vi "Configure.vi"(8 "error in (no error)":errorcluster, 11 "Autofocus in":refnum<class "Autofocus.lvclass">) -> (0 "error out":errorcluster, 2 "cancelled?":bool, 3 "Autofocus out":refnum<class "Autofocus.lvclass">)   [LabVIEW 2012, in "Autofocus.lvclass"]
doc: "The configure method configures the details for the RabbitMQ connection, the observers and the mapping script.\n\nIn the derived class, make a call to the parent for setting these parameters."
uses:
  Autofocus.lvclass
  number of subregions.ctl
  <vilib>/Utility/miscctls.llb/LVPointTypeDef.ctl
  Autofocus.lvclass/Autofocus.ctl
  <vilib>/Distrio/Murmex/Murmex/Murmex.lvclass
panel:
  in  "button::ok":bool
  in  "button::configure murmex":bool
  in  "button::cancel":bool
  in  "Tab Control":T1(tab)
  in  "Sample stage component name":string
  in  "Tomo component name":string
  in  "Camera component name":string
  in  "Focus stage component name":string
  in  "Epsilon (HC)":dbl
  in  "Epsilon (GS)":dbl
  in  "Image File Path":path
  in  "Number of subregions":T2 items=["4"=4, "5"=5]
  # "RabbitMQ parameters"
  # "Window position"
  # "Stopping parameters"
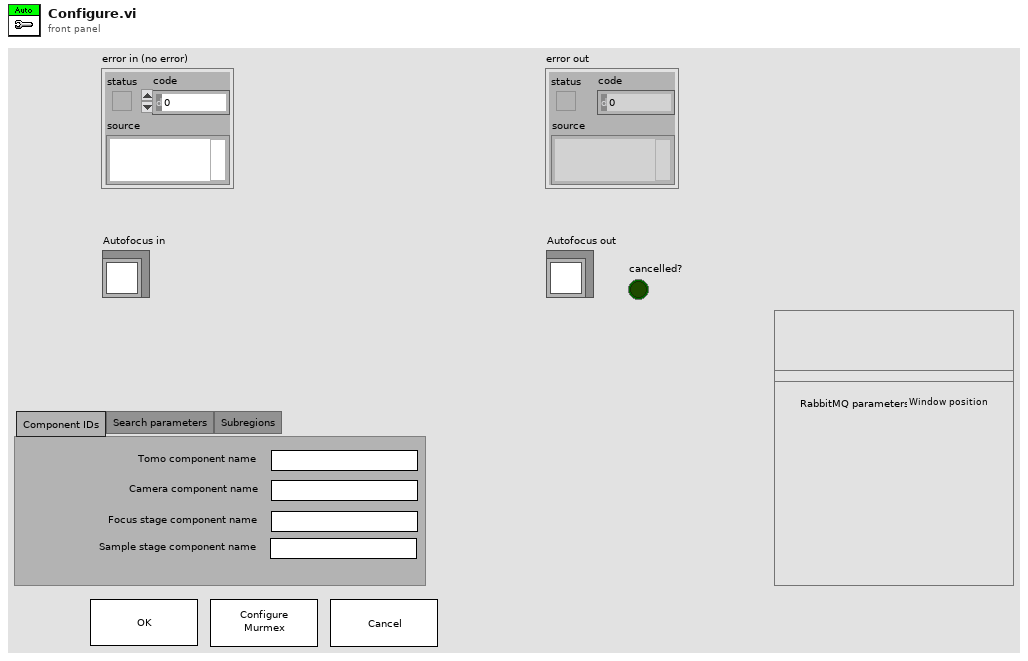
[diagram p1: front panel]
types:
  T1 = enum32{"Component IDs", "Search parameters", "Subregions"}
  T2 = typedef "Autofocus.lvclass/number of subregions.ctl" = i32
  T3 = typedef "LVPointTypeDef.ctl" = cluster{"Horizontal":i16, "Vertical":i16}
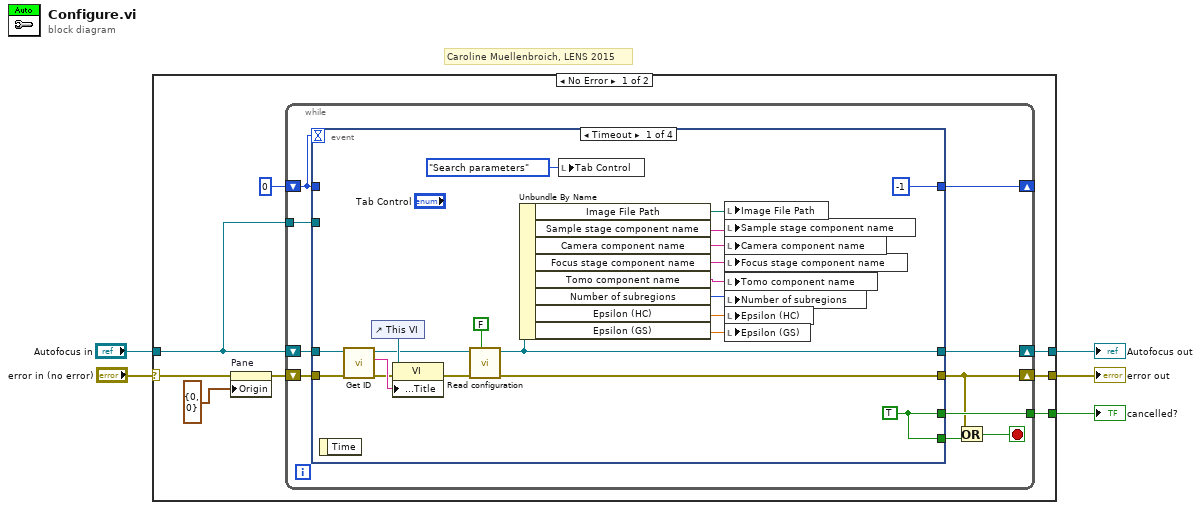
[diagram p0: block diagram]
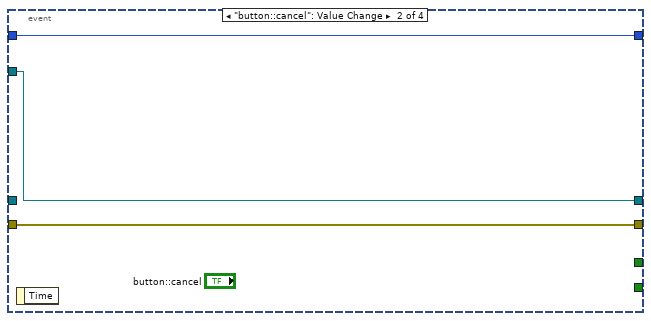
[diagram p2: hidden frame]
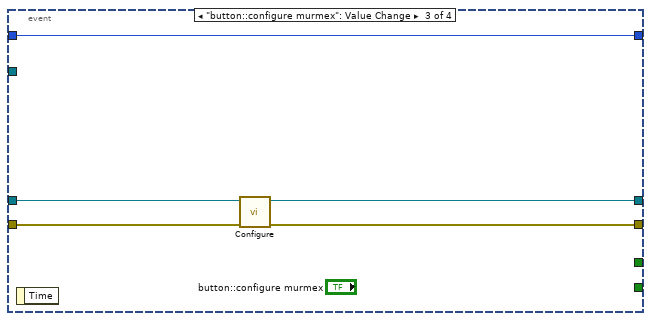
[diagram p3: hidden frame]
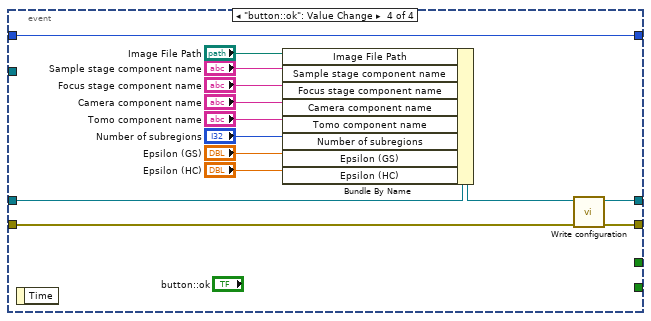
[diagram p4: hidden frame]
diagram:
  # "Caroline Muellenbroich, LENS 2015"
  n1 = case shown="No Error" "error in (no error)" {
    selector: "error in (no error)" -> [w12 w68]
    tunnel: "Autofocus in" -> [w10 w67]
    tunnel: [w8 w68] -> w3
    tunnel: [w7 w67] -> w2
    tunnel: [w6 _] -> w1
    frame No Error {
      n2 = property on="Pane" class="Pane"(error in=w12, "Origin"=T3 {"Horizontal"=0, "Vertical"=0}) -> (error out=w11:errorcluster)  [unwired: 1 in, 1 out]
      n3 = while {
        shift-right: [w18] -> w7
        shift-left: w10 -> [w20]
        shift-right: [w15] -> w8
        shift-left: w11 -> [w21]
        tunnel: w10 -> [w23]
        shift-right: [w19] -> _
        shift-left: 0 -> [w22]
        tunnel: [w17] -> w6
        stop <- w16 stop-if-true
        n4 = event shown="[0] Timeout" {
          selector: _ -> [_ _ _ _]
          dyn-events: _ -> [_ _ _ _]
          timeout: w22 -> [_ _ _ _]
          tunnel: w23 -> [_ w45 _ _]
          tunnel: w22 -> [_ w46 w48 w61]
          tunnel: w21 -> [w42 w47 w52 w64]
          tunnel: w20 -> [w41 _ w50 w63]
          tunnel: [-1 w46 w48 w61] -> w19
          tunnel: [w35 w45 w49 w65] -> w18
          tunnel: [w34 w47 w51 w66] -> w15
          tunnel: [w33 _ _ _] -> w17
          tunnel: [w33 _ _ _] -> w14
          event Timeout {
            w33 = TRUE ("force loading?")
            n5 = event-data() -> ()  [unwired: 1 in, 1 out]
            n6 = call <vilib>:"Get ID.vi"("error in (no error)"=w42, "Murmex in"=w41) -> ("error out"=w43:errorcluster, "component id"=w44:string, "Murmex out"=w38:refnum<class "Autofocus.lvclass">)  [unwired: 7 in]
            n7 = control-ref of="This VI"() -> (w40:refnum<vi>)
            n8 = property class="VI"(reference=w40, error in=w43, "Front Panel.Title"=w44) -> (error out=w39:errorcluster)  [unwired: 1 out]
            n9 = call-dynamic "Read configuration.vi"("force loading?"=FALSE, "error in (no error)"=w39, "Autofocus in"=w38) -> ("error out"=w34:errorcluster, "Autofocus out"=w35:refnum<class "Autofocus.lvclass">)  [unwired: 7 in]
            n10 = Unbundle By Name(w35) -> ("Image File Path"=w24:path, "Sample stage component name"=w25:string, "Camera component name"=w32:string, "Focus stage component name"=w31:string, "Tomo component name"=w30:string, "Number of subregions"=w29:T2, "Epsilon (HC)"=w28:dbl, "Epsilon (GS)"=w27:dbl)
            n11 = local write "Tab Control"(T1."Search parameters" ("Tab Control")) -> ()
            n12 = local write "Image File Path"(w24) -> ()
            n13 = local write "Sample stage component name"(w25) -> ()
            n14 = local write "Camera component name"(w32) -> ()
            n15 = local write "Focus stage component name"(w31) -> ()
            n16 = local write "Tomo component name"(w30) -> ()
            n17 = local write "Number of subregions"(w29) -> ()
            n18 = local write "Epsilon (HC)"(w28) -> ()
            n19 = local write "Epsilon (GS)"(w27) -> ()
          }
          event "button::cancel": Value Change {
            n20 = event-data() -> ()  [unwired: 1 in, 1 out]
          }
          event "button::configure murmex": Value Change {
            n21 = event-data() -> ()  [unwired: 1 in, 1 out]
            n22 = call-parent "Configure.vi"("error in (no error)"=w52, "Murmex in"=w50) -> ("error out"=w51:errorcluster, "Murmex out"=w49:refnum<class "Autofocus.lvclass">)  [unwired: 7 in, 1 out]
          }
          event "button::ok": Value Change {
            n23 = event-data() -> ()  [unwired: 1 in, 1 out]
            n24 = Bundle By Name(cluster=w63, "Image File Path"="Image File Path", "Sample stage component name"="Sample stage component name", "Focus stage component name"="Focus stage component name", "Camera component name"="Camera component name", "Tomo component name"="Tomo component name", "Number of subregions"="Number of subregions", "Epsilon (GS)"="Epsilon (GS)", "Epsilon (HC)"="Epsilon (HC)") -> (w62:refnum<class "Autofocus.lvclass">)
            n25 = call-dynamic "Write configuration.vi"("error in (no error)"=w64, "Autofocus in"=w62) -> ("error out"=w66:errorcluster, "Autofocus out"=w65:refnum<class "Autofocus.lvclass">)  [unwired: 8 in]
          }
        }
        n26 = Or(x=w15, y=w14) -> (x .or. y?=w16:bool)
      }
    }
    frame Error {
    }
  }
  "error out" <- w3
  "Autofocus out" <- w2
  "cancelled?" <- w1
